vi "Demo.vi"() -> ()   [LabVIEW 2017, in "LT_UpgradeFlash.lvclass"]
uses:
  LT_UpgradeFlash.lvclass
  Global.vi
panel:
  in  "show_btn":bool
  in  "selectChip_btn":bool
  in  "Close_btn":bool
  in  "Open_btn":bool
  in  "Erase_btn":bool
  in  "Read_btn":bool
  in  "chip type":u16(ring)=1 items=["LT9611", "LT6911"]
  in  "Prog_btn":bool
  out "Result String":string
  out "OK?":bool
  in  "burn file path":path=path "D:/Project/Tymphany/LT_UpgradeFlash/HDMI Board/LT FW  Files/LT9611 UXC/lt9611uxc_fw.bin"
  in  "exe path":path=path "D:/Project/Tymphany/LT_UpgradeFlash/HDMI Board/LT Upgrade Flash/Upgrade_Flash_For_Application.exe"
  in  "Stop Button":bool
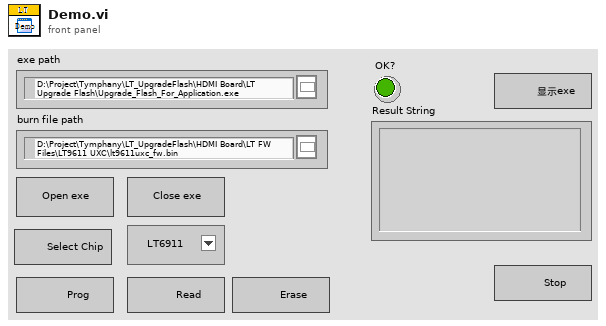
[diagram p1: front panel]
types:
  T1 = enum8{"Enabled", "Disabled", "Disabled and Grayed Out"}
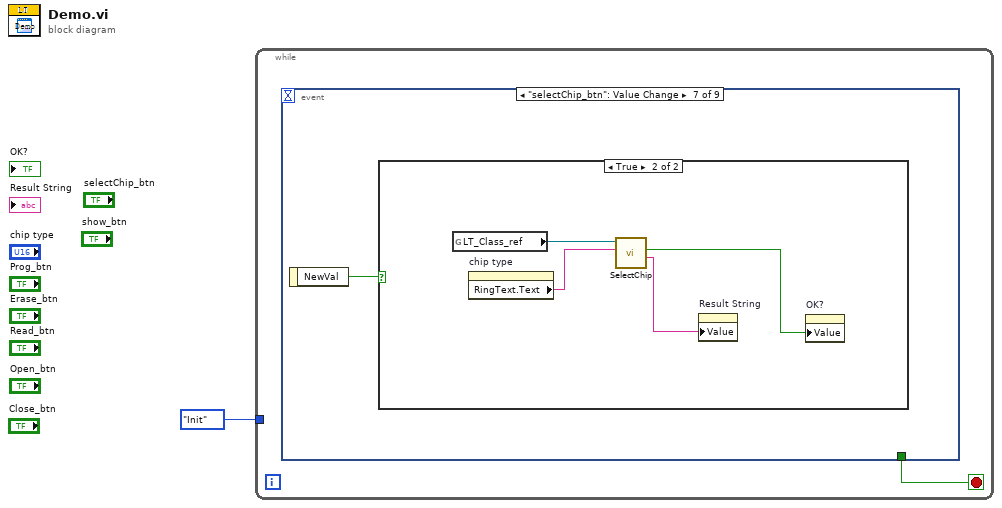
[diagram p0: block diagram]
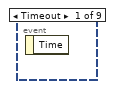
[diagram p2: hidden frame]
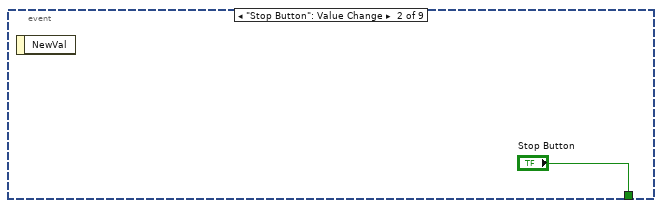
[diagram p3: hidden frame]
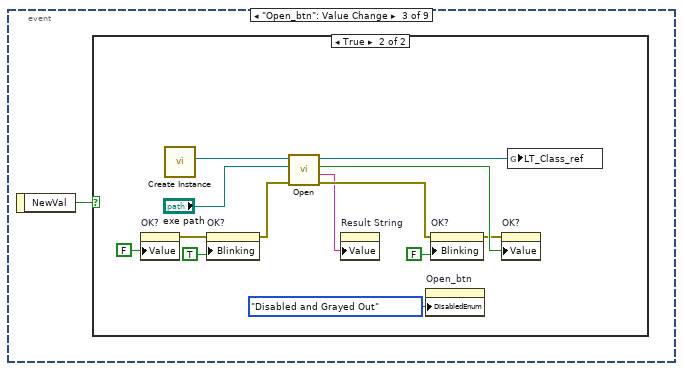
[diagram p4: hidden frame]
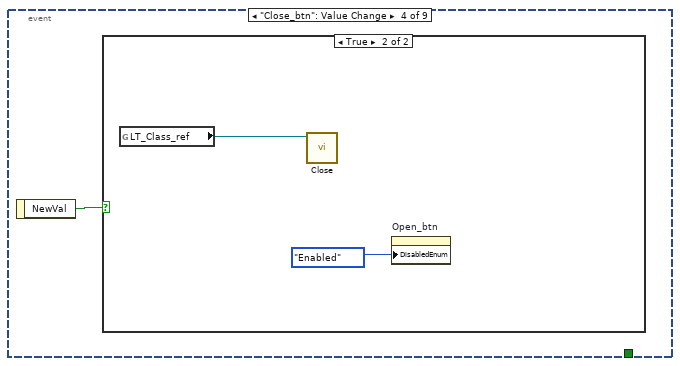
[diagram p6: hidden frame]
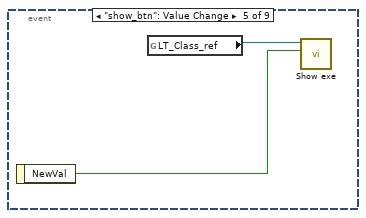
[diagram p8: hidden frame]
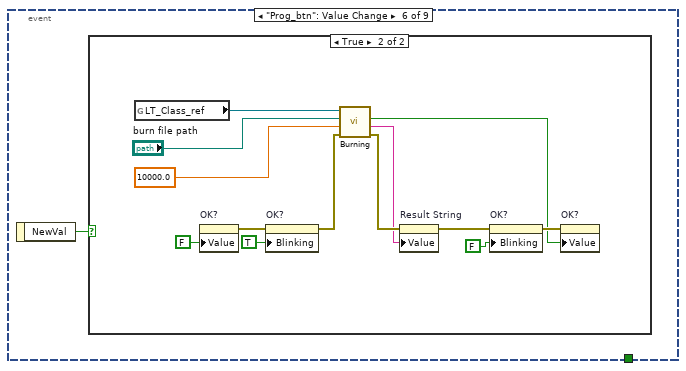
[diagram p9: hidden frame]
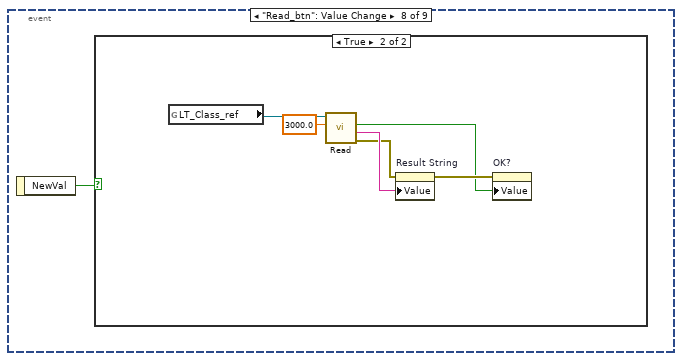
[diagram p12: hidden frame]
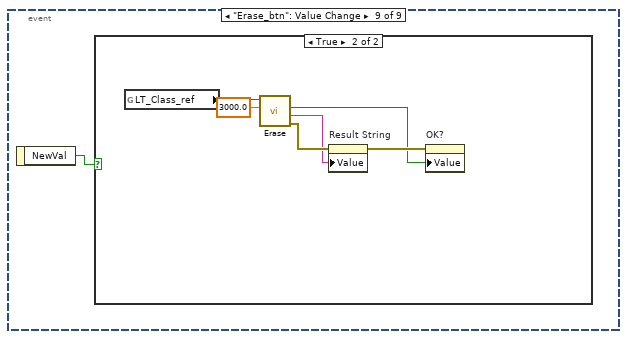
[diagram p14: hidden frame]
diagram:
  n1 = while {
    tunnel: enum16{"Init", ""}."Init" -> [_]
    stop <- w2 stop-if-true
    n2 = event shown="[6] \"selectChip_btn\": Value Change" {
      selector: _ -> [_ _ _ _ _ _ _ _ _]
      dyn-events: _ -> [_ _ _ _ _ _ _ _ _]
      timeout: _ -> [_ _ _ _ _ _ _ _ _]
      tunnel: [_ "Stop Button" _ _ _ _ _ _ _] -> w2
      event Timeout {
        n3 = event-data() -> ()  [unwired: 1 in, 1 out]
      }
      event "Stop Button": Value Change {
        n4 = event-data() -> ()  [unwired: 1 in, 1 out]
      }
      event "Open_btn": Value Change {
        n5 = event-data() -> ("NewVal"=w4:bool)  [unwired: 1 in]
        n6 = case shown="True" w4 {
          frame False {
          }
          frame True {
            n7 = property on="OK?" class="Bool (strict)"("Value"=FALSE ("OK?")) -> (error out=w13:errorcluster)  [unwired: 2 in, 1 out]
            n8 = call "Create Instance.vi"() -> ("LT_UpgradeFlash"=w15:refnum<class "LT_UpgradeFlash.lvclass">)  [unwired: 11 in]
            n9 = property on="OK?" class="Bool (strict)"(error in=w13, "Blinking"=TRUE) -> (error out=w10:errorcluster)  [unwired: 1 in, 1 out]
            n10 = call "Open.vi"("error in (no error)"=w10, "exe path"="exe path", "LT_UpgradeFlash in"=w15) -> ("error out"=w6:errorcluster, "resultStr"=w5:string, "ActionResult"=w8:bool, "LT_UpgradeFlash out"=w14:refnum<class "LT_UpgradeFlash.lvclass">)  [unwired: 5 in]
            n11 = property on="Result String" class="Str"("Value"=w5) -> ()  [unwired: 2 in, 2 out]
            n12 = property on="Open_btn" class="Bool (strict)"("DisabledEnum"=T1."Disabled and Grayed Out" ("Disabled")) -> ()  [unwired: 2 in, 2 out]
            n13 = property on="OK?" class="Bool (strict)"(error in=w6, "Blinking"=FALSE) -> (error out=w7:errorcluster)  [unwired: 1 in, 1 out]
            n14 = property on="OK?" class="Bool (strict)"(error in=w7, "Value"=w8) -> ()  [unwired: 1 in, 2 out]
            n15 = global write "Global.vi" "LT_Class_ref"(w14) -> ()
          }
        }
      }
      event "Close_btn": Value Change {
        n16 = event-data() -> ("NewVal"=w18:bool)  [unwired: 1 in]
        n17 = case shown="True" w18 {
          frame False {
          }
          frame True {
            n18 = global read "Global.vi" "LT_Class_ref"() -> (w20:refnum<class "LT_UpgradeFlash.lvclass">)
            n19 = call "Close.vi"("LT_UpgradeFlash in"=w20) -> ()  [unwired: 9 in, 2 out]
            n20 = property on="Open_btn" class="Bool (strict)"("DisabledEnum"=T1."Enabled" ("Disabled")) -> ()  [unwired: 2 in, 2 out]
          }
        }
      }
      event "show_btn": Value Change {
        n21 = event-data() -> ("NewVal"=w21:bool)  [unwired: 1 in]
        n22 = global read "Global.vi" "LT_Class_ref"() -> (w22:refnum<class "LT_UpgradeFlash.lvclass">)
        n23 = call "Show exe.vi"("show"=w21, "LT_UpgradeFlash in"=w22) -> ()  [unwired: 8 in, 2 out]
      }
      event "Prog_btn": Value Change {
        n24 = event-data() -> ("NewVal"=w23:bool)  [unwired: 1 in]
        n25 = case shown="True" w23 {
          frame False {
          }
          frame True {
            n26 = global read "Global.vi" "LT_Class_ref"() -> (w36:refnum<class "LT_UpgradeFlash.lvclass">)
            n27 = property on="OK?" class="Bool (strict)"("Value"=FALSE ("OK?")) -> (error out=w34:errorcluster)  [unwired: 2 in, 1 out]
            n28 = property on="OK?" class="Bool (strict)"(error in=w34, "Blinking"=TRUE) -> (error out=w29:errorcluster)  [unwired: 1 in, 1 out]
            n29 = call "Burning.vi"("error in (no error)"=w29, "TimeOut(s)"=10000.0 ("burning time out(ms)"), "burnFilePath"="burn file path", "LT_UpgradeFlash in"=w36) -> ("error out"=w28:errorcluster, "resultStr"=w27:string, "ActionResult"=w26:bool)  [unwired: 4 in, 1 out]
            n30 = property on="Result String" class="Str"(error in=w28, "Value"=w27) -> (error out=w25:errorcluster)  [unwired: 1 in, 1 out]
            n31 = property on="OK?" class="Bool (strict)"(error in=w25, "Blinking"=FALSE) -> (error out=w33:errorcluster)  [unwired: 1 in, 1 out]
            n32 = property on="OK?" class="Bool (strict)"(error in=w33, "Value"=w26) -> ()  [unwired: 1 in, 2 out]
          }
        }
      }
      event "selectChip_btn": Value Change {
        n33 = event-data() -> ("NewVal"=w37:bool)  [unwired: 1 in]
        n34 = case shown="True" w37 {
          frame False {
          }
          frame True {
            n35 = global read "Global.vi" "LT_Class_ref"() -> (w41:refnum<class "LT_UpgradeFlash.lvclass">)
            n36 = property on="chip type" class="Ring (strict)"() -> ("RingText.Text"=w40:string)  [unwired: 2 in, 2 out]
            n37 = call "SelectChip.vi"("chipSelection"=w40, "LT_UpgradeFlash in"=w41) -> ("resultStr"=w39:string, "ActionResult"=w38:bool)  [unwired: 6 in, 2 out]
            n38 = property on="Result String" class="Str"("Value"=w39) -> ()  [unwired: 2 in, 2 out]
            n39 = property on="OK?" class="Bool (strict)"("Value"=w38) -> ()  [unwired: 2 in, 2 out]
          }
        }
      }
      event "Read_btn": Value Change {
        n40 = event-data() -> ("NewVal"=w42:bool)  [unwired: 1 in]
        n41 = case shown="True" w42 {
          frame False {
          }
          frame True {
            n42 = global read "Global.vi" "LT_Class_ref"() -> (w48:refnum<class "LT_UpgradeFlash.lvclass">)
            n43 = call "Read.vi"("TimeOut(s)"=3000.0, "LT_UpgradeFlash in"=w48) -> ("error out"=w45:errorcluster, "resultStr"=w46:string, "ActionResult"=w44:bool)  [unwired: 6 in, 1 out]
            n44 = property on="Result String" class="Str"(error in=w45, "Value"=w46) -> (error out=w47:errorcluster)  [unwired: 1 in, 1 out]
            n45 = property on="OK?" class="Bool (strict)"(error in=w47, "Value"=w44) -> ()  [unwired: 1 in, 2 out]
          }
        }
      }
      event "Erase_btn": Value Change {
        n46 = event-data() -> ("NewVal"=w49:bool)  [unwired: 1 in]
        n47 = case shown="True" w49 {
          frame False {
          }
          frame True {
            n48 = global read "Global.vi" "LT_Class_ref"() -> (w55:refnum<class "LT_UpgradeFlash.lvclass">)
            n49 = call "Erase.vi"("timeOut(ms)"=3000.0, "LT_UpgradeFlash in"=w55) -> ("error out"=w53:errorcluster, "resultStr"=w52:string, "ActionResult"=w51:bool)  [unwired: 6 in, 1 out]
            n50 = property on="Result String" class="Str"(error in=w53, "Value"=w52) -> (error out=w54:errorcluster)  [unwired: 1 in, 1 out]
            n51 = property on="OK?" class="Bool (strict)"(error in=w54, "Value"=w51) -> ()  [unwired: 1 in, 2 out]
          }
        }
      }
    }
  }
